vi "Get All Package Versions.vi"(7 "LabVIEW Web Service Request":refnum<class "Web Request.lvclass">) -> ()   [LabVIEW 2016]
uses:
  <vilib>/wsapi/Web Request.lvclass
  Libraries/Packages/Repo_class/Repo.lvclass/Repo.ctl
  Libraries/Packages/Package_class/Package.lvclass/Package.ctl
  Libraries/Packages/Package_class/Read Versions.vi
  Libraries/Packages/Package_class/Read Name.vi
  Libraries/Packages/Repo_class/Read Packages.vi
  <vilib>/addons/JSON API/JSON Array/JSON Array.lvclass
  C:/Program Files (x86)/National Instruments/LabVIEW 2016/vi.lib/addons/JSON API/JSON Value/JSON Value.lvclass
  Libraries/WSsupport/GV_Repos.vi
  <vilib>/addons/JSON API/JSON Value/JSON Value.lvclass
  Libraries/Packages/Package_class/Package.lvclass
  Libraries/Packages/Package Version_class/Package Version.lvclass
  Libraries/WSsupport/WSsupport.lvlib
  Libraries/ServerErrors/ServerErrors.lvlib
  Libraries/Packages/Repo_class/Repo.lvclass
panel:
  # "Use the Web Service Request input terminal to call the VIs on the Web Services palette. Do not remove it from the connector pane unless you don't need access to the palette."
  # "Each additional control wired to the connector pane will be available as an input in the URL. To include an indicator in terminal-mode output (the default setting), it must also be wired to the connector pane."
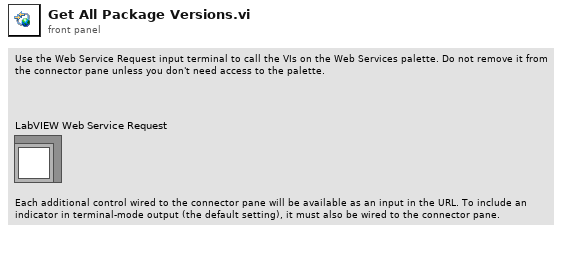
[diagram p1: front panel]
types:
  T1 = typedef "ServerErrors.lvlib/Error Message--cluster.ctl" = cluster{"HTTP Code":i32, "JSON Response":cluster{"error":string, "reason":string}}
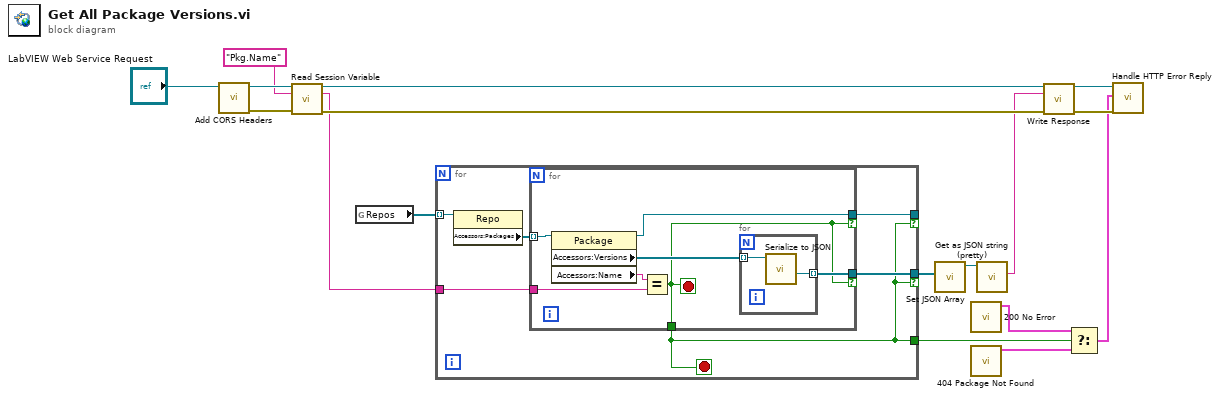
[diagram p0: block diagram]
diagram:
  n1 = call "Add CORS Headers.vi"("LabVIEW Web Service Request"="LabVIEW Web Service Request") -> ("error out"=w15:errorcluster, "LabVIEW Web Service Request out"=w16:refnum<class "Web Request.lvclass">)  [unwired: 9 in]
  n2 = call <vilib>:"Read Session Variable.vi"("LabVIEW Web Service Request"=w16, "key"="Pkg.Name", "error in (no error)"=w15) -> ("LabVIEW Web Service Request out"=w13:refnum<class "Web Request.lvclass">, "value"=w10:string, "error out"=w12:errorcluster)  [unwired: 10 in]
  n3 = global read "GV_Repos.vi" "Repos"() -> (w11:refnum<class "Repo.lvclass">[])
  n4 = for {
    tunnel: w11 -> [w23] mode=indexing
    tunnel: w10 -> [w21]
    tunnel: [w20] -> _ if=w18
    tunnel: [w18] -> w7
    tunnel: [w19] -> w3 if=w18
    stop <- w18 stop-if-true
    n5 = property class="Repo"(reference=w23) -> ("Accessors:Packages"=w22:refnum<class "Package.lvclass">[])  [unwired: 1 in, 2 out]
    n6 = for {
      tunnel: w22 -> [w30] mode=indexing
      tunnel: w21 -> [w28]
      tunnel: [w24] -> w18
      tunnel: [w27] -> w20 if=w24
      tunnel: [w25] -> w19 if=w24
      stop <- w24 stop-if-true
      n7 = property class="Package"(reference=w30) -> (reference out=w27:refnum<class "Package.lvclass">, "Accessors:Versions"=w26:refnum<class "Package Version.lvclass">[], "Accessors:Name"=w29:string)  [unwired: 1 in, 1 out]
      n8 = Equal?(x=w29, y=w28) -> (x = y?=w24:bool)
      n9 = for {
        tunnel: w26 -> [w32] mode=indexing
        tunnel: [w31] -> w25 mode=indexing
        n10 = call-dynamic "Serialize to JSON.vi"("Pkg Details in"=w32) -> ("JSON Value"=w31:refnum<class "JSON Value.lvclass">)  [unwired: 7 in, 3 out]
      }
    }
  }
  n11 = call <vilib>:"Set JSON Array.vi"("Array"=w3) -> ("JSON Array out"=w2:refnum<class "JSON Array.lvclass">)  [unwired: 9 in, 1 out]
  n12 = call "200 No Error.vi"() -> ("no error"=w4:T1)  [unwired: 11 in]
  n13 = call "404 Package Not Found.vi"() -> ("error"=w6:T1)  [unwired: 11 in]
  n14 = call <vilib>:"Get as JSON string (pretty).vi"("JSON Value in"=w2) -> ("<JSON>"=w1:string)  [unwired: 9 in, 1 out]
  n15 = call <vilib>:"Write Response.vi"("LabVIEW Web Service Request"=w13, "response string"=w1, "error in (no error)"=w12) -> ("LabVIEW Web Service Request out"=w9:refnum<class "Web Request.lvclass">, "error out"=w8:errorcluster)  [unwired: 11 in]
  n16 = Select(t=w4, s=w7, f=w6) -> (s? t:f=w5:T1)
  n17 = call "Handle HTTP Error Reply.vi"("error in (no error)"=w8, "HTTP Status Code"=w5, "Web Request in"=w9) -> ()  [unwired: 8 in, 1 out]
